vi "M01 Wind Turbine.vi"(11 "NXT/EV3":T1) -> (1 "Angle out":sgl=47.0, 3 "EV3 out":T1)   [LabVIEW 2016]
uses:
  <vilib>/NXT/Subs/LVHSConnector.ctl
  <vilib>/NXT/LegoClasses/BrickReference/BrickReference.lvclass
  <vilib>/NXT/Dual Mode Library/Waits/Wait_Num.vi
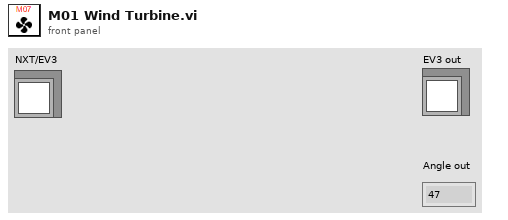
[diagram p1: front panel]
types:
  T1 = typedef "LVHSConnector.ctl" = refnum<class "BrickReference.lvclass">
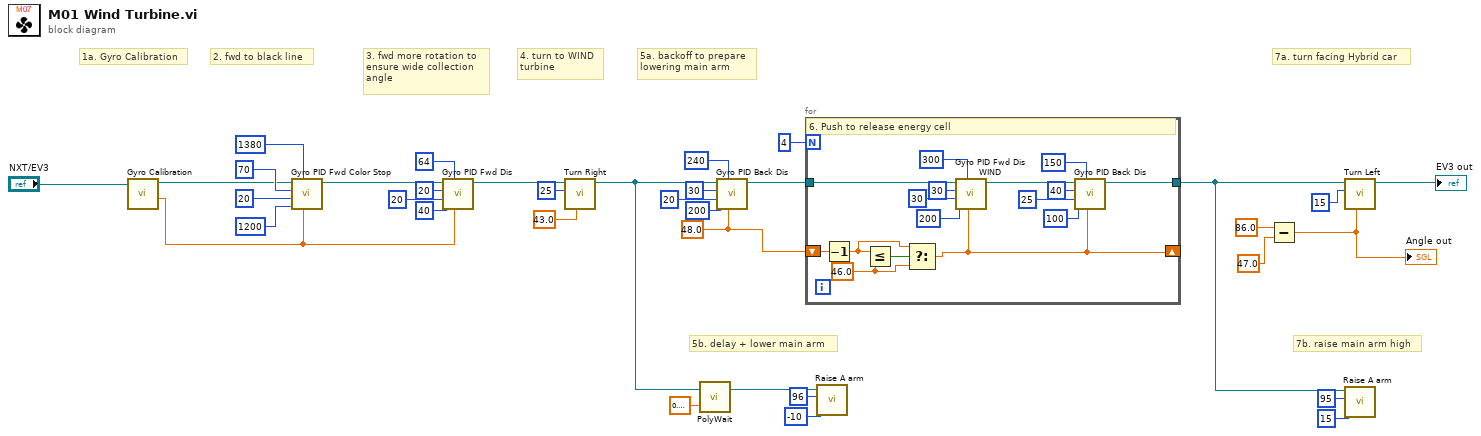
[diagram p0: block diagram]
diagram:
  w2 = sgl 48.0 ("Ini. Degrees")
  # "7b. raise main arm high"
  # "7a. turn facing Hybrid car"
  # "5b. delay + lower main arm"
  # "5a. backoff to prepare\nlowering main arm"
  # "4. turn to WIND\nturbine"
  # "3. fwd more rotation to\nensure wide collection\nangle"
  # "2. fwd to black line"
  # "1a. Gyro Calibration"
  n1 = call "Gyro Calibration.vi"("NXT/EV3"="NXT/EV3") -> ("Degrees"=w28:sgl, "NXT/EV3"=w15:T1)  [unwired: 6 in, 1 out]
  n2 = call "Gyro PID Fwd Color Stop.vi"("Target angle"=w28, "Threshold to Color"=1380 ("Threshold to C1"), "Threshold to slow"=1200 ("Threshold to De-acc"), "Min. speed"=20 ("De-acc"), "Max. speed"=70 ("Acc"), "EV3 in"=w15) -> ("EV3 out"=w32:T1)  [unwired: 5 in]
  n3 = call "Gyro PID Fwd Dis.vi"("Target angle"=w28, "Threshold to stop"=64 ("Stop rotation"), "Threshold to slow"=40 ("Threshold to De-acc"), "Min. speed"=20 ("De-acc"), "Max. speed"=20 ("Acc"), "EV3 in"=w32) -> ("EV3 out"=w27:T1)  [unwired: 5 in]
  n4 = call "Turn Right.vi"("Turning angle"=sgl 43.0, "Motor B (right)"=i8 25, "EV3 in"=w27) -> ("EV3 out"=w11:T1)  [unwired: 8 in]
  n5 = call-poly <vilib>:"PolyWait.vi"("Time (1 sec)"=sgl 0.3, "NXT/EV3"=w11) -> ("NXT/EV3"=w6:T1)  [unwired: 2 in]
  n6 = call "Gyro PID Back Dis.vi"("Target angle"=w2, "Threshold to stop"=240 ("Stop rotation"), "Threshold to slow"=200 ("Threshold to De-acc"), "Min. speed"=20 ("De-acc"), "Max. speed"=30 ("Acc"), "EV3 in"=w11) -> ("EV3 out"=w10:T1)  [unwired: 5 in]
  n7 = for {
    N: 4 -> [_]
    tunnel: w10 -> [w43]
    tunnel: [w42] -> w3
    shift-right: [w36] -> _
    shift-left: w2 -> [w40]
    w37 = sgl 46.0 ("y")
    # "6. Push to release energy cell"
    n8 = Decrement(x=w40) -> (x-1=w38:sgl)
    n9 = Less Or Equal?(x=w38, y=w37) -> (x <= y?=w39:bool)
    n10 = Select(t=w38, s=w39, f=w37) -> (s? t:f=w36:sgl)
    n11 = call "Gyro PID Fwd Dis WIND.vi"("Target angle"=w36, "Threshold to stop"=300 ("Stop rotation"), "Threshold to slow"=200 ("Threshold to De-acc"), "Higher speed"=30 ("De-acc"), "Max. speed"=30 ("Acc"), "EV3 in"=w43) -> ("EV3 out"=w44:T1)  [unwired: 5 in]
    n12 = call "Gyro PID Back Dis.vi"("Target angle"=w36, "Threshold to stop"=150 ("Stop rotation"), "Threshold to slow"=100 ("Threshold to De-acc"), "Min. speed"=25 ("De-acc"), "Max. speed"=40 ("Acc"), "EV3 in"=w44) -> ("EV3 out"=w42:T1)  [unwired: 5 in]
  }
  n13 = call "Raise A arm.vi"("Power"=i8 -10, "Rotation"=96, "EV3 in"=w6) -> ()  [unwired: 8 in, 1 out]
  n14 = Subtract(x=86.0, y=47.0) -> (x-y=w18:dbl)
  "Angle out" <- w18
  n15 = call "Turn Left.vi"("Turning angle"=w18, "Motor B (right)"=i8 15, "EV3 in"=w3) -> ("EV3 out"=→"EV3 out":T1)  [unwired: 8 in]
  n16 = call "Raise A arm.vi"("Power"=i8 15, "Rotation"=95, "EV3 in"=w3) -> ()  [unwired: 8 in, 1 out]
